vi "Cleanup.vi"(8 "error in (no error)":errorcluster, 11 "Device in":refnum<class "Device.lvclass">) -> (0 "error out":errorcluster)   [LabVIEW 2020, in "HAL.lvlib" / "Device.lvclass"]
uses:
  Device.lvclass
  Device.lvclass/Device.ctl
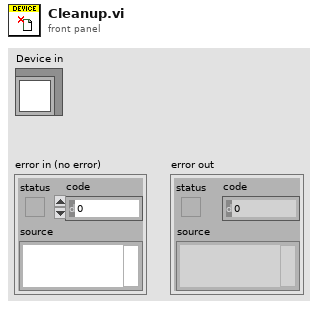
[diagram p1: front panel]
types:
  T1 = typedef "HAL.lvlib/Device.lvclass/Ref Data.ctl" = cluster{"Config Keys":string[], "Config Values":string[], "Cal Expires":timestamp, "Name":string, "Comment":string, "State":T2, "Error":errorcluster}
  T2 = typedef "HAL.lvlib/Device.lvclass/Device State.ctl" = enum16{"Uninitialized", "Initialized", "Configured", "Running", "Error"}
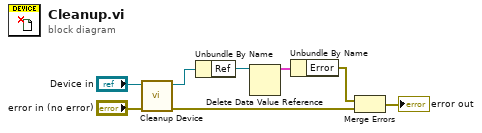
[diagram p0: block diagram]
diagram:
  n1 = call-dynamic "Cleanup Device.vi"("error in (no error)"="error in (no error)", "Device in"="Device in") -> ("error out"=w6:errorcluster, "Device out"=w5:refnum<class "Device.lvclass">)  [unwired: 8 in]
  n2 = Unbundle By Name(w5) -> ("Ref"=w4:refnum<data-value>)
  n3 = Delete Data Value Reference(data value reference=w4) -> (data value=w3:T1)  [unwired: 1 in, 1 out]
  n4 = Unbundle By Name(w3) -> ("Error"=w1:errorcluster)
  n5 = Merge Errors(w1, w6) -> (→"error out":errorcluster)
